vi "DebugControl_Provider_OnPopupMenu.vi"(11 "objects":T1[](array[typedef])) -> ()   [LabVIEW 2018]
uses:
  <resource>/Framework/Providers/API/ItemRef.ctl
  <resource>/Framework/Providers/API/mxLvMenuItem.ctl
panel:
  out "error out":errorcluster
  in  "error in":errorcluster
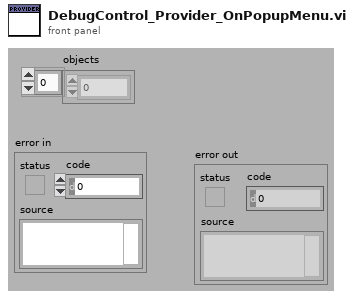
[diagram p1: front panel]
types:
  T1 = typedef "ItemRef.ctl" = u64
  T2 = typedef "mxLvMenuItem.ctl" = cluster{"Menu Name":string, "Description":string, "Icon File Name":path, "Menu Tag":string, "Enabled":bool, "Checked":bool, "Separator":bool, "Batchable":bool, "Weight":i32, "Batch Mode (Ignored if Not Batchable)":enum32{"Show If All Items Support Command", "Show If Any Items Support Command"}, "Menu Location":enum32{"<None>", "Project", "Project / Build Specifications", "Tools", "Tools / Source Control", "Tools / Real-Time Module", "Help"}, "Exclude From Getting Started Window Menu":bool}
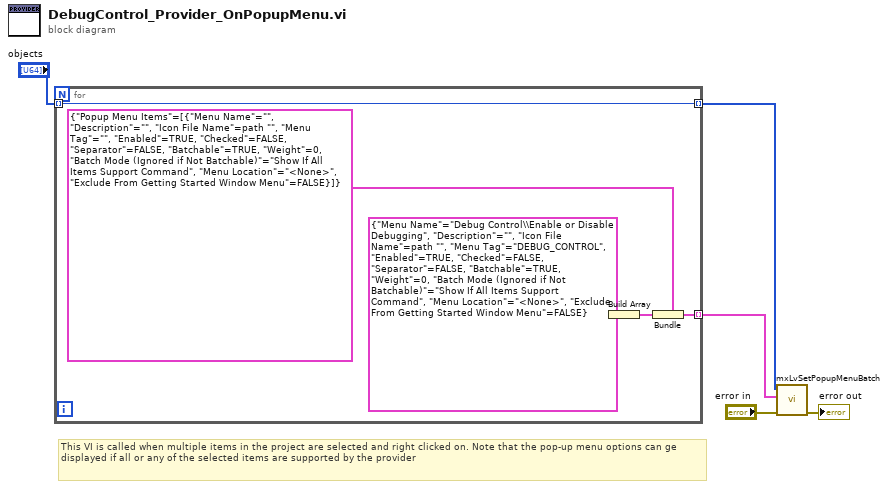
[diagram p0: block diagram]
diagram:
  # "This VI is called when multiple items in the project are selected and right clicked on. Note that the pop-up menu options can ge displayed if all or any of the selected items are supported by the provider"
  n1 = for {
    tunnel: [w8] -> w5 mode=indexing
    tunnel: "objects" -> [w6] mode=indexing
    tunnel: [w6] -> w1 mode=indexing
    n2 = Build Array(T2 {"Menu Name"="Debug Control\\Enable or Disable Debugging", "Description"="", "Icon File Name"=path "", "Menu Tag"="DEBUG_CONTROL", "Enabled"=TRUE, "Checked"=FALSE, "Separator"=FALSE, "Batchable"=TRUE, "Weight"=0, "Batch Mode (Ignored if Not Batchable)"=enum."Show If All Items Support Command", "Menu Location"=enum."<None>", "Exclude From Getting Started Window Menu"=FALSE} ("Menu Item")) -> (w9:T2[])
    n3 = Bundle(cluster=cluster{"Popup Menu Items":T2[]} {"Popup Menu Items"=[{"Menu Name"="", "Description"="", "Icon File Name"=path "", "Menu Tag"="", "Enabled"=TRUE, "Checked"=FALSE, "Separator"=FALSE, "Batchable"=TRUE, "Weight"=0, "Batch Mode (Ignored if Not Batchable)"=enum."Show If All Items Support Command", "Menu Location"=enum."<None>", "Exclude From Getting Started Window Menu"=FALSE}]}, "Popup Menu Items"=w9) -> (w8:cluster{"Popup Menu Items":T2[]})
  }
  n4 = call <resource>:"mxLvSetPopupMenuBatch.vi"("error in"="error in", "Menu Items"=w5, "Items"=w1) -> ("error out"=→"error out":errorcluster)  [unwired: 7 in, 1 out]
